vi "extractPressureData.vi"(8 "error in (no error)":errorcluster, 11 "ILC in":refnum<class "ILC.lvclass">) -> (0 "error out":errorcluster, 3 "ILC out":refnum<class "ILC.lvclass">)   [LabVIEW 2015, in "ILCCommon.lvlib" / "ILC.lvclass"]
uses:
  <userlib>/Common/ILC/ILC/ILC.lvclass
  <userlib>/Common/ILC/ILCModelTypedefs/FinalDelimiter.ctl
  <userlib>/Common/ILC/ILC/ILC.lvclass/ILC.ctl
  <userlib>/Common/ILC/ILCModelTypedefs/ILCModelTypedefs.lvlib
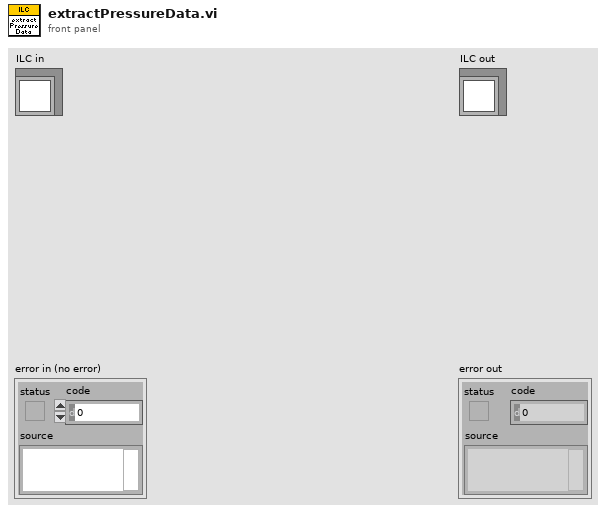
[diagram p1: front panel]
types:
  T1 = typedef "ILCCommon.lvlib/ILCModelTypedefs.lvlib/FinalDelimiter.ctl" = enum16{",", "<CR><LF>"}
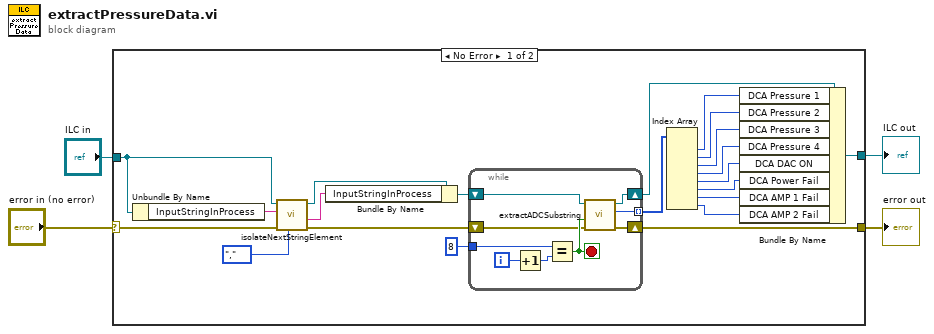
[diagram p0: block diagram]
diagram:
  n1 = case shown="No Error" "error in (no error)" {
    selector: "error in (no error)" -> [w8 w36]
    tunnel: [w18 w36] -> w3
    tunnel: [w24 w35] -> w1
    tunnel: "ILC in" -> [w10 w35]
    frame No Error {
      n2 = Unbundle By Name(w10) -> ("InputStringInProcess"=w12:string)
      n3 = call <userlib>:"isolateNextStringElement.vi"("Final Delimiter"=FinalDelimiter.",", "error in (no error)"=w8, "inputString"=w12, "ILC in"=w10) -> ("error out"=w7:errorcluster, "remainingString"=w6:string, "ILC out"=w9:refnum<class "ILC.lvclass">)  [unwired: 4 in, 1 out]
      n4 = Bundle By Name(cluster=w9, "InputStringInProcess"=w6) -> (w11:refnum<class "ILC.lvclass">)
      n5 = while {
        tunnel: 8 -> [w30]
        tunnel: [w28] -> w23 mode=indexing
        shift-right: [w27] -> w18
        shift-left: w7 -> [w26]
        shift-right: [w34] -> w25
        shift-left: w11 -> [w33]
        i -> [w32]
        stop <- w29 stop-if-true
        n6 = Increment(x=w32) -> (x+1=w31:i32)
        n7 = Equal?(x=w30, y=w31) -> (x = y?=w29:bool)
        n8 = call <userlib>:"extractADCSubstring.vi"("error in (no error)"=w26, "lastIsTrue?"=w29, "ILC in"=w33) -> ("error out"=w27:errorcluster, "adcElement"=w28:i32, "ILC out"=w34:refnum<class "ILC.lvclass">)  [unwired: 6 in]
      }
      n9 = Index Array(array=w23) -> (element #1=w22:i32, element #2=w21:i32, element #3=w20:i32, element #4=w19:i32, element #5=w16:i32, element #6=w15:i32, element #7=w14:i32, element #8=w13:i32)  [unwired: 8 in]
      n10 = Bundle By Name(cluster=w25, "DCA Pressure 1"=w22, "DCA Pressure 2"=w21, "DCA Pressure 3"=w20, "DCA Pressure 4"=w19, "DCA DAC ON"=w16, "DCA Power Fail"=w15, "DCA AMP 1 Fail"=w14, "DCA AMP 2 Fail"=w13) -> (w24:refnum<class "ILC.lvclass">)
    }
    frame Error {
    }
  }
  "error out" <- w3
  "ILC out" <- w1
